vi "Initialize.vi"(6 "optional":variant, 8 "error in":errorcluster, 11 "xceDataNode in":refnum<class "xceDataNode.lvclass">) -> (0 "error out":errorcluster, 3 "Node*":refnum<data-value>)   [LabVIEW 2013, in "xceDataNode.lvclass"]
doc: "Initializes a node. Makes a data value reference of the node, sets the selfNode, and output the data value reference."
uses:
  xceDataNode.lvclass
  xceNode/xceNode.lvclass
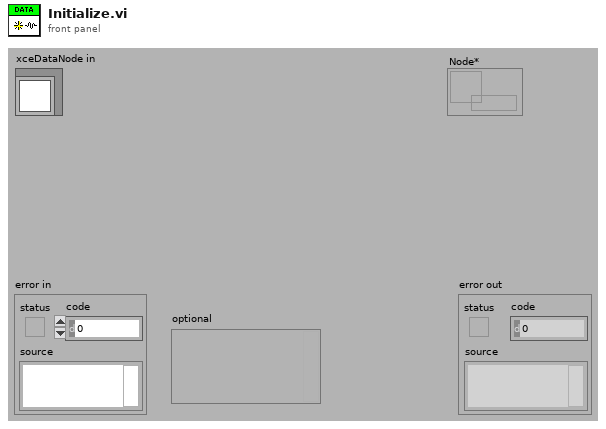
[diagram p1: front panel]
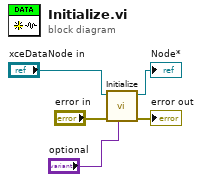
[diagram p0: block diagram]
diagram:
  n1 = call-parent "Initialize.vi"("optional"="optional", "error in"="error in", "xceNode in"="xceDataNode in") -> ("error out"=→"error out":errorcluster, "Node*"=→"Node*":refnum<data-value>)  [unwired: 7 in]
